vi "Configure Display Data.vi"(0 "VISA resource name":refnum<visa-resource-name>, 5 "Interval (4 : 1min)":i32(ring)=4 items=["5 seconds", "10 seconds", "15 seconds", "30 seconds", "1 minute", "2 minutes", "5 minutes", "10 minutes", "15 minutes", "20 minutes", "30 minutes", "1 hour", "2 hours", "4 hours", "10 hours"], 7 "File Save Interval (3 : 1hour)":i32(ring)=3 items=["10 minutes", "20 minutes", "30 minutes", "1 hour", "2 hours", "3 hours", "4 hours", "6 hours", "8 hours", "12 hours", "1 day", "2 days", "3 days", "5 days", "7 days", "14 days", "31 days"], 11 "error in (no error)":errorcluster) -> (4 "VISA resource name out":refnum<visa-resource-name>, 15 "error out":errorcluster)   [LabVIEW 2020, in "Yokogawa GX Series.lvlib"]
doc: "Sets the display data recording mode.\n\nCommand: SDispData"
uses:
  <instrlib>/Yokogawa GX Series/Yokogawa GX Series.lvlib
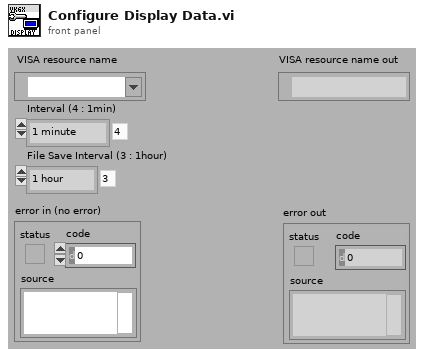
[diagram p1: front panel]
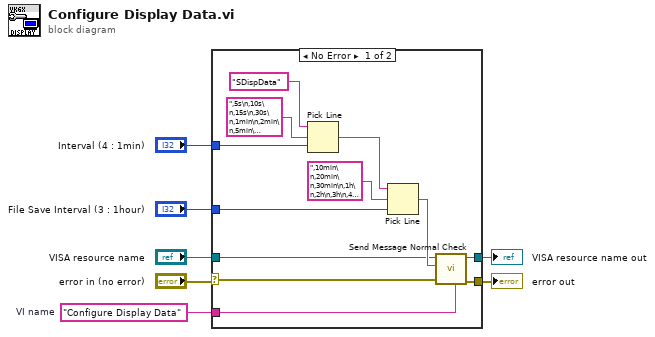
[diagram p0: block diagram]
diagram:
  w6 = "Configure Display Data"  # VI name
  n1 = case shown="No Error" "error in (no error)" {
    selector: "error in (no error)" -> [w8 w20]
    tunnel: "File Save Interval (3 : 1hour)" -> [w17 _]
    tunnel: w6 -> [w16 _]
    tunnel: "Interval (4 : 1min)" -> [w14 _]
    tunnel: [w13 w21] -> w4
    tunnel: [w12 w20] -> w3
    tunnel: "VISA resource name" -> [w9 w21]
    frame No Error {
      n2 = Pick Line(string ("")="SDispData", multi-line string=",5s\n,10s\n,15s\n,30s\n,1min\n,2min\n,5min\n,10min\n,15min\n,20min\n,30min\n,1h\n,2h\n,4h\n,10h", line index=w14) -> (output string=w15:string)
      n3 = Pick Line(string ("")=w15, multi-line string=",10min\n,20min\n,30min\n,1h\n,2h\n,3h\n,4h\n,6h\n,8h\n,12h\n,1Day\n,2Day\n,3Day\n,5Day\n,7Day\n,14Day\n,31Day", line index=w17) -> (output string=w18:string)
      n4 = call <instrlib>:"Send Message Normal Check.vi"("Source (\"\")"=w16, "error in (no error)"=w8, "Send Message (\"\")"=w18, "VISA resource name"=w9) -> ("error out"=w12:errorcluster, "VISA resource name out"=w13:refnum<visa-resource-name>)  [unwired: 2 in, 4 out]
    }
    frame Error {
    }
  }
  "error out" <- w3
  "VISA resource name out" <- w4
